vi "ReadAllCtlRefs_Core.vi"(8 "error in (no error)":errorcluster, 11 "ctlrRef_VAT in":refnum<class "ctlRef_VAT.lvclass">) -> (0 "error out":errorcluster, 1 "Values":refnum<vi>[](array[refnum]), 2 "Names":string[](array[string]), 3 "ctlrRef_VAT out":refnum<class "ctlRef_VAT.lvclass">)   [LabVIEW 2020, in "CtlReferences.lvlib" / "ctlRef_VAT.lvclass"]
uses:
  ctlRef_VAT.lvclass
  ctlRef_VAT.lvclass/ctlRef_VAT.ctl
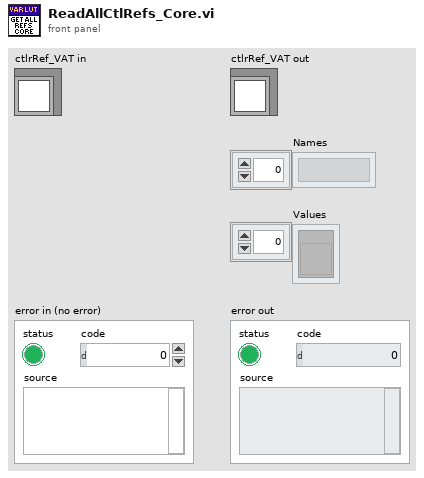
[diagram p1: front panel]
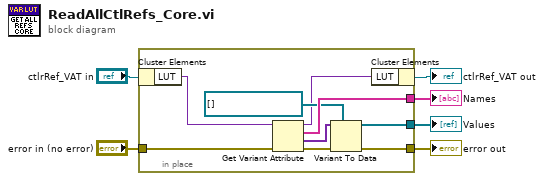
[diagram p0: block diagram]
diagram:
  n1 = in-place {
    in-place-border: [w15] -> w4
    in-place-border: [w10] -> w3
    in-place-border: [w12] -> w2
    in-place-border: "error in (no error)" -> [w8]
    n2 = in-place-cluster #1("ctlrRef_VAT in") -> ("LUT"=w13:variant)
    n3 = Get Variant Attribute(Variant=w13, error in=w8) -> (duplicate Variant=w7:variant, names=w15:string[], values=w11:variant[], error out=w14:errorcluster)  [unwired: 2 in]
    n4 = Variant To Data(error in=w14, type=refnum<vi>[] [], Variant=w11) -> (data=w10:refnum<vi>[], error out=w12:errorcluster)
    n5 = in-place-cluster #1("LUT"=w7) -> (→"ctlrRef_VAT out":refnum<class "ctlRef_VAT.lvclass">)
  }
  "error out" <- w2
  "Values" <- w3
  "Names" <- w4
